vi "Teleop.vi"(10 "Match Info":T1={"Autonomous Elapsed Seconds"=0.0, "TeleOp Elapsed Seconds"=0.0, "Disabled Elapsed Seconds"=0.0, "Visited Autonomous"=FALSE, "Visited TeleOp"=FALSE, "Visited Disabled"=FALSE, "Autonomous Settings"={"Autonomous Style"=enum."Independent", "VI Refnum"=refnum}}, 11 "Call Context":T2) -> ()   [LabVIEW 2016]
doc: "This VI is called for each TeleOp packet received from the DS where the robot is not disabled. It is often used to read from the joysticks and update I/O or to update setpoints for timed control loops. It should complete and return within 20 milliseconds or it may miss DS packets."
uses:
  <vilib>/Rock Robotics/WPI/DriverStation/WPI_DriverStationDerivedRobotMode.ctl
  <vilib>/Rock Robotics/WPI/DriverStation/WPI_DriverStationMatch Info.ctl
  <vilib>/Rock Robotics/WPI/Utilities/WPI_GetSetVariantRefNum.vi
  <vilib>/Rock Robotics/Network Tables/NT Read Boolean.vi
  <vilib>/Rock Robotics/Network Tables/NT Read Number.vi
  <vilib>/Rock Robotics/Network Tables/NT Write Numeric Array.vi
  <vilib>/Rock Robotics/Network Tables/NT Write Boolean Array.vi
  <vilib>/Rock Robotics/Network Tables/NT Write Number.vi
  Robot Global Data.vi
  <vilib>/Rock Robotics/WPI/Ultrasonic/WPI_UltrasonicRangeUnits.ctl
  <vilib>/Rock Robotics/WPI/Ultrasonic/WPI_SonarSRF04DigitalRefNum Registry Get.vi
  <vilib>/Rock Robotics/WPI/Ultrasonic/WPI_SonarSRF04DigitalGetRange.vi
  <vilib>/Rock Robotics/WPI/RobotDrive/WPI_RobotDriveMecanumDrive_Cartesian.vi
panel:
  out "Numeric 2":dbl
  out "Numeric":dbl
  out "Sample Slider 0":dbl(slide) scale=0.0..5.0
  out "Sample Boolean 1":bool
  out "Sample Boolean 0":bool
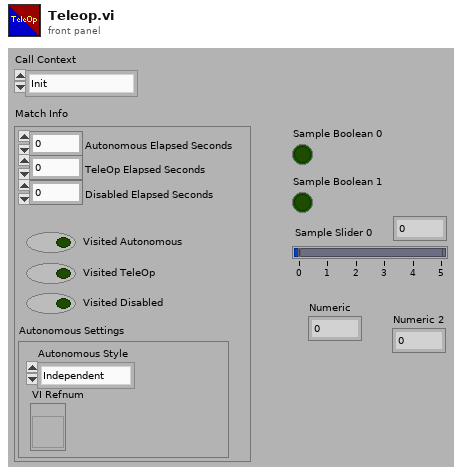
[diagram p1: front panel]
types:
  T1 = typedef "WPI_DriverStationMatch Info.ctl" = cluster{"Autonomous Elapsed Seconds":dbl, "TeleOp Elapsed Seconds":dbl, "Disabled Elapsed Seconds":dbl, "Visited Autonomous":bool, "Visited TeleOp":bool, "Visited Disabled":bool, "Autonomous Settings":cluster{"Autonomous Style":enum16{"Iterative", "Independent"}, "VI Refnum":refnum<vi>}}
  T2 = typedef "WPI_DriverStationDerivedRobotMode.ctl" = enum16{"Init", "Execute", "Stop"}
  T3 = typedef "WPI_JoystickDevRef.ctl" = cluster{"Device":T4}
  T4 = typedef "WPI_JoystickDeviceEnum.ctl" = enum16{"USB 0", "USB 1", "USB 2", "USB 3", "USB 4", "USB 5"}
  T5 = typedef "WPI_MotorControlDeviceRef.ctl" = cluster{"DeviceStatus":errorcluster, "Type":T6, "PWM":cluster{"PWM Channel":T7, "DeadBand":T8}, "CAN":cluster{"Device Number":u8, "SetOutput VI Ref":variant, "GetOutput VI Ref":variant, "Enable VI Ref":variant, "Disable VI Ref":variant, "Data":variant}, "Invert":bool}
  T6 = typedef "WPI_MotorControlType.ctl" = enum16{"PWM", "CAN"}
  T7 = typedef "FPGA_DIOPWMChannel.ctl" = enum8{"PWM 0", "PWM 1", "PWM 2", "PWM 3", "PWM 4", "PWM 5", "PWM 6", "PWM 7", "PWM 8", "PWM 9", "PWM MXP 0", "PWM MXP 1", "PWM MXP 2", "PWM MXP 3", "PWM MXP 4", "PWM MXP 5", "PWM MXP 6", "PWM MXP 7", "PWM MXP 8", "PWM MXP 9", "Invalid"}
  T8 = typedef "WPI_PWMDeadband.ctl" = cluster{"Name":string, "maxPositivePwm":i32, "minPositivePwm":i32, "centerPwm":i32, "maxNegativePwm":i32, "minNegativePwm":i32, "angularRange":u16}
  T9 = typedef "WPI_RelayDevRef.ctl" = cluster{"DevStatus":errorcluster, "Relay Channel":T10, "Relay Direction":T11}
  T10 = typedef "FPGA_DIORelayChannel.ctl" = enum8{"Relay 0", "Relay 1", "Relay 2", "Relay 3", "Invalid"}
  T11 = typedef "WPI_RelayDirection.ctl" = enum16{"Both directions", "Forward only", "Reverse only"}
  T12 = typedef "WPI_UltrasonicRangeUnits.ctl" = enum16{"inches", "mm"}
  T13 = typedef "WPI_UltrasonicDeviceRef.ctl" = cluster{"DevStatus":errorcluster, "Ping Channel":T14, "Echo Channel":T14, "CntIndex":T15}
  T14 = typedef "FPGA_DIOChannel.ctl" = enum8{"DIO 0", "DIO 1", "DIO 2", "DIO 3", "DIO 4", "DIO 5", "DIO 6", "DIO 7", "DIO 8", "DIO 9", "DIO MXP 0", "DIO MXP 1", "DIO MXP 2", "DIO MXP 3", "DIO MXP 4", "DIO MXP 5", "DIO MXP 6", "DIO MXP 7", "DIO MXP 8", "DIO MXP 9", "DIO MXP 10", "DIO MXP 11", "DIO MXP 12", "DIO MXP 13", "DIO MXP 14", "DIO MXP 15", "SPI Port CS1", "SPI Port CS2", "SPI Port CS3", "SPI Port MISO", "SPI Port MOSI", "Invalid"}
  T15 = typedef "FPGA_CounterCtrSystemIndex.ctl" = enum8{"Ctr 0", "Ctr 1", "Ctr 2", "Ctr 3", "Ctr 4", "Ctr 5", "Ctr 6", "Ctr 7", "Invalid"}
  T16 = typedef "WPI_EncoderDevRef.ctl" = cluster{"DevStatus":errorcluster, "EncoderIndex":T17, "CounterIndex":T15, "DistancePerCount":dbl, "Decoding Type":T18}
  T17 = typedef "FPGA_EncoderIdx.ctl" = enum8{"Enc 0", "Enc 1", "Enc 2", "Enc 3", "Enc 4", "Enc 5", "Enc 6", "Enc 7", "Invalid"}
  T18 = typedef "WPI_EncoderType.ctl" = enum16{"1x", "2x", "4x"}
  T19 = typedef "WPI_RobotDriveDevRef.ctl" = cluster{"DevStatus":errorcluster, "Motors[]":T5[], "Square Inputs":bool, "Max Output":dbl}
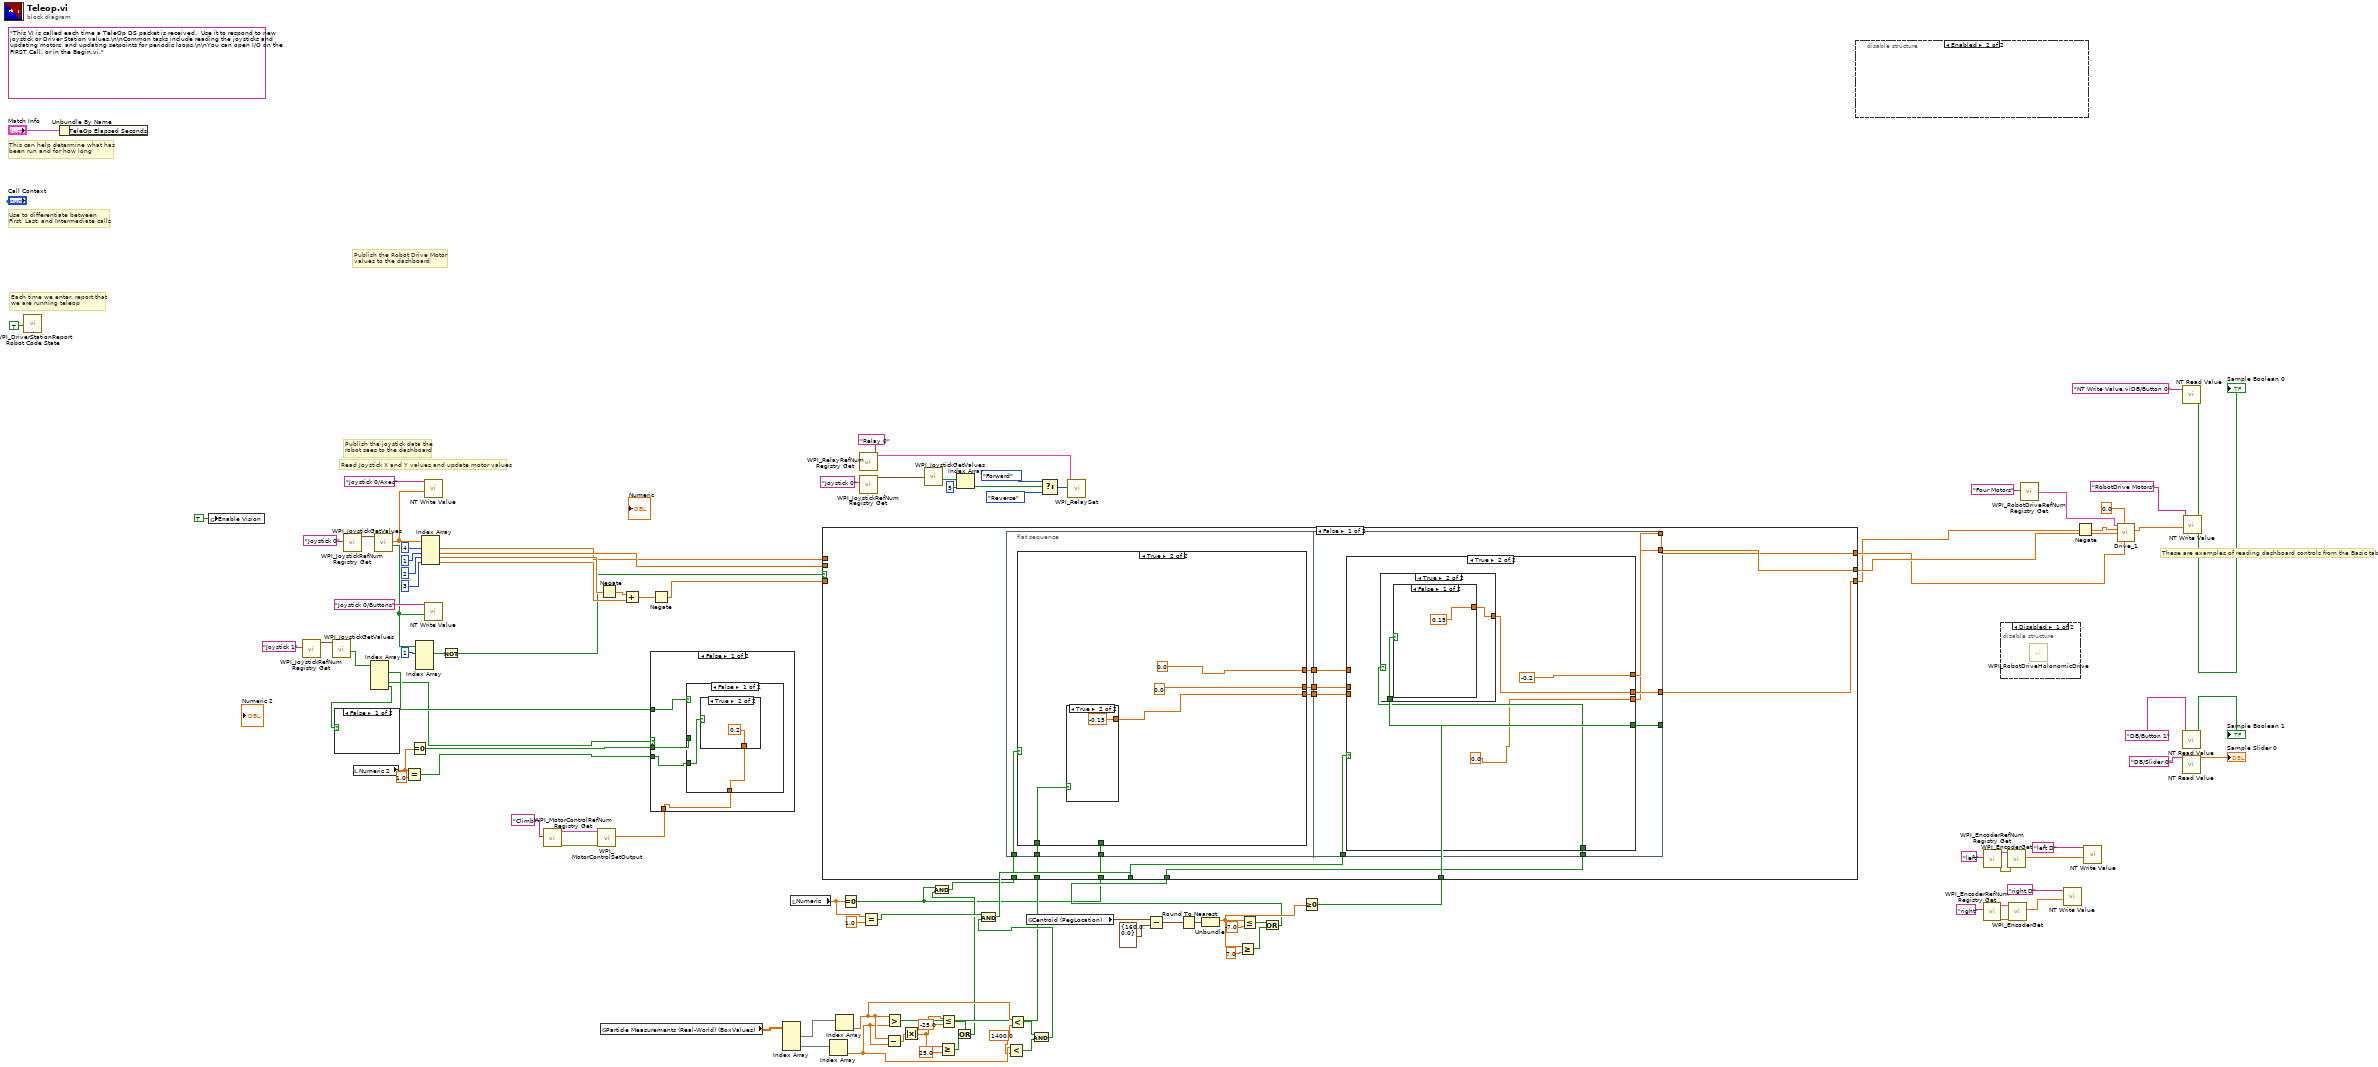
[diagram p0: block diagram]
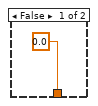
[diagram p3: hidden frame]
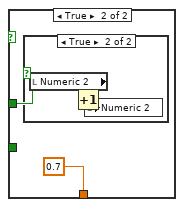
[diagram p4: hidden frame]
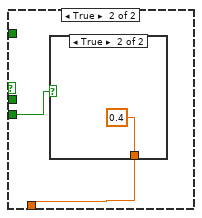
[diagram p6: hidden frame]
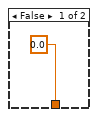
[diagram p7: hidden frame]
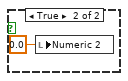
[diagram p8: hidden frame]
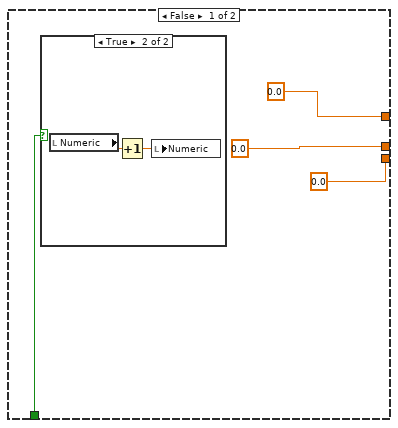
[diagram p9: hidden frame]
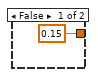
[diagram p11: hidden frame]
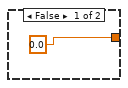
[diagram p13: hidden frame]
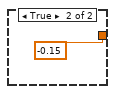
[diagram p14: hidden frame]
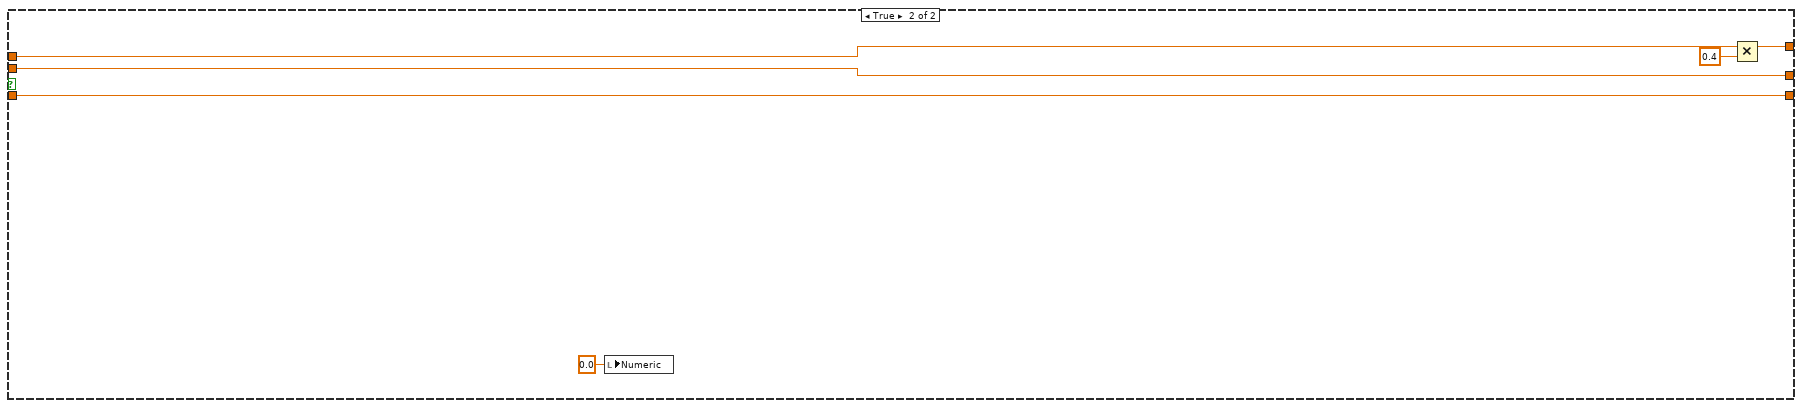
[diagram p15: hidden frame]
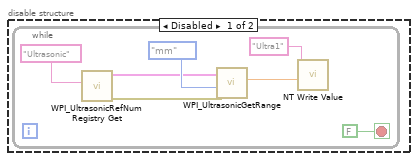
[diagram p16: hidden frame]
diagram:
  w59 = 1400.0
  (unwired) "This VI is called each time a TeleOp DS packet is received.  Use it to respond to new joystick or Driver Station values.\n\nCommon tasks include reading the joysticks and updating motors, and updating setpoints for periodic loops.\n\nYou can open I/O on the FIRST Call, or in the Begin.vi."
  # "These are examples of reading dashboard controls from the Basic tab"
  # "Publish the Robot Drive Motor\nvalues to the dashboard"
  # "Publish the joystick data the\nrobot sees to the dashboard"
  # "Each time we enter, report that\nwe are running teleop"
  # "Use to differentiate between\nFirst, Last, and Intermediate calls"
  # "This can help determine what has\nbeen run and for how long"
  # "Read Joystick X and Y values and update motor values"
  n1 = call <vilib>:"WPI_DriverStationReport Robot Code State.vi"("TeleOp"=TRUE ("Autonomous")) -> ()  [unwired: 10 in, 1 out]
  n2 = Unbundle By Name("Match Info") -> ()  [unwired: 1 out]
  n3 = global write "Robot Global Data.vi" "Enable Vision"(TRUE ("Enable Vision")) -> ()
  n4 = call <vilib>:"WPI_JoystickRefNum Registry Get.vi"("refnum name"="Joystick 1") -> ("JoystickDevRef"=w27:T3)  [unwired: 1 in, 9 out]
  n5 = call <vilib>:"WPI_JoystickGetValues.vi"("JoystickDevRef"=w27) -> ("Buttons"=w25:bool[])  [unwired: 6 in, 4 out]
  n6 = call <vilib>:"WPI_JoystickRefNum Registry Get.vi"("refnum name"="Joystick 0") -> ("JoystickDevRef"=w104:T3)  [unwired: 1 in, 9 out]
  n7 = local read "Numeric 2"() -> (w29:dbl)
  n8 = Index Array(array=w25) -> (element #1=w24:bool, element #3=w22:bool, element #4=w23:bool)  [unwired: 4 in, 1 out]
  n9 = case shown="False" w23 {
    frame False {
    }
    frame True {
      n10 = local write "Numeric 2"(0.0 ("Numeric 2")) -> ()
    }
  }
  n11 = call <vilib>:"WPI_JoystickGetValues.vi"("JoystickDevRef"=w104) -> ("Buttons"=w19:bool[], "Axes"=w92:dbl[])  [unwired: 6 in, 3 out]
  n12 = Equal?(x=w29, y=1.0) -> (x = y?=w21:bool)
  n13 = Equal To 0?(x=w29) -> (x = 0?=w28:bool)
  n14 = Index Array(array=w19, index #1=1 ("index")) -> (element #1=w73:bool)  [unwired: 3 in, 3 out]
  n15 = Index Array(array=w92, index #1=4 ("index"), index #2=1 ("index"), index #3=2 ("index"), index #4=3 ("index")) -> (element #1=w20:dbl, element #2=w71:dbl, element #3=w91:dbl, element #4=w89:dbl)
  n16 = call-poly <vilib>:"NT Write Value.vi"("Numeric Array"=w92, "Name"="Joystick 0/Axes") -> ()  [unwired: 9 in, 1 out]
  n17 = call-poly <vilib>:"NT Write Value.vi"("Boolean Array"=w19, "Name"="Joystick 0/Buttons") -> ()  [unwired: 9 in, 1 out]
  n18 = Not(x=w73) -> (.not. x?=w44:bool)
  n19 = call <vilib>:"WPI_MotorControlRefNum Registry Get.vi"("refnum name"="Climb") -> ("error out"=w41:errorcluster, "MotorControlDevRef"=w42:T5)  [unwired: 9 in]
  n20 = Negate(x=w91) -> (-x=w90:dbl)
  n21 = global read "Robot Global Data.vi" "Particle Measurements (Real-World) (BoxValues)"() -> (w69:dbl[][])
  n22 = Add(x=w90, y=w89) -> (x+y=w78:dbl)
  n23 = case shown="False" w22 {
    tunnel: [w110 w120] -> w40
    tunnel: w28 -> [w111 _]
    tunnel: w24 -> [w109 _]
    tunnel: w21 -> [w108 w121]
    frame False {
      n24 = case shown="False" w109 {
        tunnel: [w113 0.7] -> w110
        tunnel: w108 -> [w112 _]
        tunnel: w111 -> [_ w116]
        frame False {
          n25 = case shown="True" w112 {
            tunnel: [0.0 0.2] -> w113
            frame False {
            }
            frame True {
            }
          }
        }
        frame True {
          n26 = case shown="True" w116 {
            frame False {
            }
            frame True {
              n27 = local read "Numeric 2"() -> (w119:dbl)
              n28 = Increment(x=w119) -> (x+1=w118:dbl)
              n29 = local write "Numeric 2"(w118) -> ()
            }
          }
        }
      }
    }
    frame True {
      n30 = case shown="True" w121 {
        tunnel: [0.0 ("y") 0.4 ("y")] -> w120
        frame False {
        }
        frame True {
        }
      }
    }
  }
  n31 = call <vilib>:"WPI_MotorControlSetOutput.vi"("error in (no error)"=w41, "Output"=w40, "MotorControlDevRef"=w42) -> ()  [unwired: 6 in, 3 out]
  n32 = Negate(x=w78) -> (-x=w70:dbl)
  n33 = Index Array(array=w69) -> (element #1=w68:dbl[], element #2=w67:dbl[])  [unwired: 4 in]
  n34 = local read "Numeric"() -> (w38:dbl)
  n35 = Index Array(array=w67) -> (element=w60:dbl)  [unwired: 1 in]
  n36 = Index Array(array=w68) -> (element=w61:dbl)  [unwired: 1 in]
  n37 = Equal To 0?(x=w38) -> (x = 0?=w32:bool)
  n38 = call <vilib>:"WPI_RelayRefNum Registry Get.vi"("refnum name"="Relay 0") -> ("RelayDevRef"=w6:T9)  [unwired: 9 in, 1 out]
  n39 = call <vilib>:"WPI_JoystickRefNum Registry Get.vi"("refnum name"="Joystick 0") -> ("JoystickDevRef"=w10:T3)  [unwired: 9 in, 1 out]
  n40 = Equal?(x=w38, y=1.0) -> (x = y?=w37:bool)
  n41 = Subtract(x=w61, y=w60) -> (x-y=w66:dbl)
  n42 = Greater?(x=w61, y=w60) -> (0:w34:bool)
  n43 = Absolute Value(x=w66) -> (abs(x)=w56:dbl)
  n44 = call <vilib>:"WPI_JoystickGetValues.vi"("JoystickDevRef"=w10) -> ("Buttons"=w9:bool[])  [unwired: 6 in, 4 out]
  n45 = Greater Or Equal?(x=w56, y=25.0) -> (x >= y?=w63:bool)
  n46 = Less Or Equal?(x=w56, y=-25.0) -> (x <= y?=w62:bool)
  n47 = Or(x=w62, y=w63) -> (x .or. y?=w33:bool)
  n48 = And(x=w32, y=w33) -> (x .and. y?=w31:bool)
  n49 = Index Array(array=w9, index=5) -> (element=w1:bool)
  n50 = Less?(x=w60, y=w59) -> (x < y?=w57:bool)
  n51 = Less?(x=w61, y=w59) -> (x < y?=w58:bool)
  n52 = global read "Robot Global Data.vi" "Centroid (PegLocation)"() -> (w49:cluster{"X Centroid":sgl, "Y Centroid":sgl})
  n53 = And(x=w58, y=w57) -> (x .and. y?=w36:bool)
  n54 = And(x=w37, y=w36) -> (x .and. y?=w35:bool)
  n55 = Select(t=enum16{"Off", "On", "Forward", "Reverse"}."Forward", s=w1, f=enum16{"Off", "On", "Forward", "Reverse"}."Reverse") -> (s? t:f=w3:enum16{"Off", "On", "Forward", "Reverse"})
  n56 = call <vilib>:"WPI_RelaySet.vi"("RelayValue"=w3, "RelayDevRef"=w6) -> ()  [unwired: 8 in, 2 out]
  n57 = Subtract(x=w49, y=cluster{"X Centroid":sgl, "Y Centroid":sgl} {"X Centroid"=160.0, "Y Centroid"=0.0}) -> (x-y=w50:cluster{"X Centroid":sgl, "Y Centroid":sgl})
  n58 = Round To Nearest(number=w50) -> (nearest integer value=w55:cluster{"X Centroid":sgl, "Y Centroid":sgl})
  n59 = Unbundle(w55) -> ("X Centroid"=w47:sgl)  [unwired: 1 out]
  n60 = Greater Or Equal?(x=w47, y=sgl 7.0) -> (x >= y?=w53:bool)
  n61 = Less Or Equal?(x=w47, y=sgl -7.0 ("x")) -> (x <= y?=w54:bool)
  n62 = Or(x=w54, y=w53) -> (x .or. y?=w46:bool)
  n63 = Greater Or Equal To 0?(x=w47) -> (x >= 0?=w45:bool)
  n64 = case shown="False" w44 {
    tunnel: w20 -> [_ w181]
    tunnel: [w132 w177] -> w13
    tunnel: w71 -> [_ w180]
    tunnel: [w134 w180] -> w16
    tunnel: w70 -> [_ w179]
    tunnel: [w133 w179] -> w12
    tunnel: w46 -> [w131 _]
    tunnel: w45 -> [w135 _]
    tunnel: w35 -> [w130 _]
    tunnel: w32 -> [w126 _]
    tunnel: w34 -> [w125 _]
    tunnel: w31 -> [w124 _]
    frame False {
      n65 = flat-sequence {
        tunnel: [w141] -> w129
        tunnel: [w140] -> w128
        tunnel: [w139] -> w127
        tunnel: w126 -> [w138]
        tunnel: w125 -> [w137]
        tunnel: w124 -> [w136]
        tunnel: w135 -> [w162]
        tunnel: [w161] -> w134
        tunnel: [w160] -> w133
        tunnel: [w159] -> w132
        tunnel: w131 -> [w158]
        tunnel: w130 -> [w157]
        tunnel: w129 -> [w156]
        tunnel: w128 -> [w155]
        tunnel: w127 -> [w154]
        frame #0 {
          n66 = case shown="True" w136 {
            tunnel: [0.0 0.0] -> w140
            tunnel: [0.0 0.0] -> w141
            tunnel: [0.0 w149] -> w139
            tunnel: w138 -> [w142 _]
            tunnel: w137 -> [_ w148]
            frame False {
              n67 = case shown="True" w142 {
                frame False {
                }
                frame True {
                  n68 = local read "Numeric"() -> (w147:dbl)
                  n69 = Increment(x=w147) -> (x+1=w146:dbl)
                  n70 = local write "Numeric"(w146) -> ()
                }
              }
            }
            frame True {
              n71 = case shown="True" w148 {
                tunnel: [0.15 -0.15] -> w149
                frame False {
                }
                frame True {
                }
              }
            }
          }
        }
        frame #1 {
          n72 = case shown="True" w157 {
            tunnel: [w164 w167] -> w160
            tunnel: [w165 -0.2] -> w161
            tunnel: [w163 0.0] -> w159
            tunnel: w158 -> [_ w168]
            tunnel: w162 -> [_ w169]
            tunnel: w156 -> [w165 _]
            tunnel: w155 -> [w164 _]
            tunnel: w154 -> [w163 _]
            frame False {
            }
            frame True {
              n73 = case shown="True" w168 {
                tunnel: [0.0 w173] -> w167
                tunnel: w169 -> [_ w172]
                frame False {
                }
                frame True {
                  n74 = case shown="False" w172 {
                    tunnel: [0.15 -0.15] -> w173
                    frame False {
                    }
                    frame True {
                    }
                  }
                }
              }
            }
          }
        }
      }
    }
    frame True {
      n75 = local write "Numeric"(0.0 ("Numeric")) -> ()
      n76 = Multiply(x=w181, y=0.4) -> (x*y=w177:dbl)
    }
  }
  n77 = disable-structure shown="Enabled" {
    frame Disabled {
      n78 = while {
        stop <- FALSE stop-if-true
        n79 = call-poly <vilib>:"WPI_UltrasonicRefNum Registry Get.vi"("refnum name"="Ultrasonic") -> ("error out"=w183:errorcluster, "SonarSRF04DevRef"=w184:T13)  [unwired: 9 in]
        n80 = call-poly <vilib>:"WPI_UltrasonicGetRange.vi"("error in (no error)"=w183, "Range Units"=WPI_UltrasonicRangeUnits."mm", "SonarSRF04DevRef"=w184) -> ("Distance"=w187:dbl)  [unwired: 6 in, 2 out]
        n81 = call-poly <vilib>:"NT Write Value.vi"("Numeric"=w187, "Name"="Ultra1") -> ()  [unwired: 9 in, 1 out]
      }
    }
    frame Enabled {
    }
  }
  n82 = call <vilib>:"WPI_EncoderRefNum Registry Get.vi"("refnum name"="right") -> ("error out"=w86:errorcluster, "EncoderDevRef"=w85:T16)  [unwired: 9 in]
  n83 = call <vilib>:"WPI_EncoderRefNum Registry Get.vi"("refnum name"="left") -> ("error out"=w88:errorcluster, "EncoderDevRef"=w87:T16)  [unwired: 9 in]
  n84 = disable-structure shown="Disabled" {
    frame Disabled {
      n85 = call-poly <vilib>:"WPI_RobotDriveHolonomicDrive.vi"() -> ()  [unwired: 9 in, 3 out]
    }
    frame Enabled {
    }
  }
  n86 = call <vilib>:"WPI_EncoderGet.vi"("error in (no error)"=w88, "EncoderDevRef"=w87) -> ("Distance"=w80:dbl)  [unwired: 4 in, 5 out]
  n87 = call <vilib>:"WPI_EncoderGet.vi"("error in (no error)"=w86, "EncoderDevRef"=w85) -> ("Distance"=w79:dbl)  [unwired: 4 in, 5 out]
  n88 = call <vilib>:"WPI_RobotDriveRefNum Registry Get.vi"("refnum name"="Four Motors") -> ("RobotDriveDevRef"=w17:T19)  [unwired: 1 in, 9 out]
  n89 = call-poly <vilib>:"NT Write Value.vi"("Numeric"=w79, "Name"="right D") -> ()  [unwired: 9 in, 1 out]
  n90 = Negate(x=w12) -> (-x=w11:dbl)
  n91 = call-poly <vilib>:"NT Write Value.vi"("Numeric"=w80, "Name"="left D") -> ()  [unwired: 9 in, 1 out]
  n92 = call "Drive_1.vi"("Rotation"=w13, "Gyro Angle"=0.0, "Y"=w16, "X"=w11, "RobotDriveDevRef 2"=w17) -> ("Motor Values"=w15:dbl[])  [unwired: 4 in, 2 out]
  n93 = call-poly <vilib>:"NT Read Value.vi"("Name"="NT Write Value.viDB/Button 0" ("refnum name")) -> ("Boolean"=→"Sample Boolean 0":bool)  [unwired: 9 in, 1 out]
  n94 = call-poly <vilib>:"NT Read Value.vi"("Name"="DB/Button 1" ("refnum name")) -> ("Boolean"=→"Sample Boolean 1":bool)  [unwired: 9 in, 1 out]
  n95 = call-poly <vilib>:"NT Read Value.vi"("Name"="DB/Slider 0" ("refnum name")) -> ("Numeric"=→"Sample Slider 0":dbl)  [unwired: 9 in, 1 out]
  n96 = call-poly <vilib>:"NT Write Value.vi"("Numeric Array"=w15, "Name"="RobotDrive Motors") -> ()  [unwired: 9 in, 1 out]
